vi "filter_array (subVI).vi"(8 "filter":bool[](array[boolean]), 11 "array":dbl[](array[numeric])) -> (3 "filtered array":dbl[](array[numeric]))   [LabVIEW 2021]
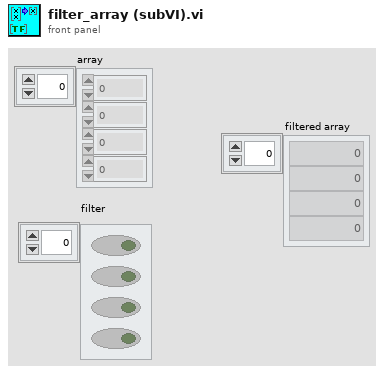
[diagram p1: front panel]
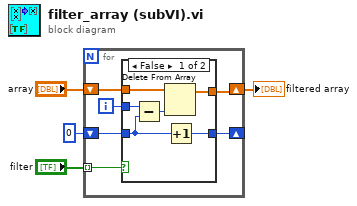
[diagram p0: block diagram]
diagram:
  n1 = for {
    tunnel: "filter" -> [w10] mode=indexing
    shift-right: [w7] -> w1
    shift-left: "array" -> [w9]
    shift-right: [w5] -> _
    shift-left: 0 -> [w6]
    i -> [w8]
    n2 = case shown="False" w10 {
      tunnel: w9 -> [w16 w18]
      tunnel: w8 -> [w15 _]
      tunnel: [w14 w18] -> w7
      tunnel: w6 -> [w12 w17]
      tunnel: [w11 w17] -> w5
      frame False {
        n3 = Subtract(x=w15, y=w12) -> (x-y=w13:i32)
        n4 = Delete From Array(array=w16, index=w13) -> (array with subset deleted=w14:dbl[])  [unwired: 1 in, 1 out]
        n5 = Increment(x=w12) -> (x+1=w11:i32)
      }
      frame True {
      }
    }
  }
  "filtered array" <- w1
